vi "Calculate Driving Direction.vi"(9 "obstacle distance":dbl=0.4, 10 "IRData":T1[](array[typedef]), 11 "velocity in":T2) -> (3 "velocity out":T2)   [LabVIEW 2014]
uses:
  <vilib>/robotics/TaimiOmni/TaimiOmni/TaimiOmniVelocity.ctl
  <vilib>/robotics/TaimiOmni/TaimiOmni/TaimiOmniIRData.ctl
  <vilib>/Analysis/baseanly.llb/Real Dot Product.vi
  <vilib>/Analysis/NI_AALBase.lvlib
  <vilib>/robotics/TaimiOmni/TaimiOmni/TaimiOmni.lvclass
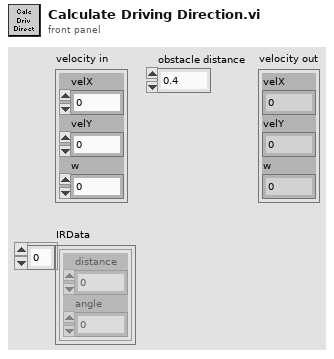
[diagram p1: front panel]
types:
  T1 = typedef "TaimiOmni.lvclass/TaimiOmniIRData.ctl" = cluster{"distance":dbl, "angle":dbl}
  T2 = typedef "TaimiOmni.lvclass/TaimiOmniVelocity.ctl" = cluster{"velX":dbl, "velY":dbl, "w":dbl}
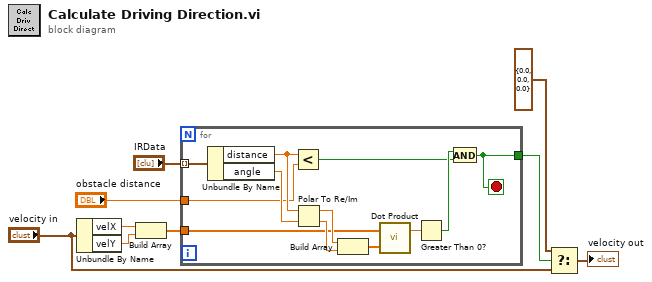
[diagram p0: block diagram]
diagram:
  n1 = Unbundle By Name("velocity in") -> ("velX"=w8:dbl, "velY"=w7:dbl)
  n2 = Build Array(w8, w7) -> (w6:dbl[])
  n3 = for {
    tunnel: "IRData" -> [w21] mode=indexing
    tunnel: w6 -> [w17]
    tunnel: "obstacle distance" -> [w13]
    tunnel: [w10] -> w4
    stop <- w10 stop-if-true
    n4 = Unbundle By Name(w21) -> ("distance"=w14:dbl, "angle"=w20:dbl)
    n5 = Less?(x=w14, y=w13) -> (x < y?=w11:bool)
    n6 = Polar To Re/Im(2:w20, 3:w14) -> (0:w18:dbl, 1:w19:dbl)
    n7 = Build Array(w19, w18) -> (w16:dbl[])
    n8 = call-poly <vilib>:"Dot Product.vi"("Y Vector"=w16, "X Vector"=w17) -> ("X * Y"=w15:dbl)  [unwired: 1 out]
    n9 = Greater Than 0?(x=w15) -> (x > 0?=w12:bool)
    n10 = And(x=w12, y=w11) -> (x .and. y?=w10:bool)
  }
  n11 = Select(t=T2 {"velX"=0.0, "velY"=0.0, "w"=0.0}, s=w4, f="velocity in") -> (s? t:f=→"velocity out":T2)
